vi "Check if File Exists _NOT Folder.vi"(8 "error in (no error)":errorcluster, 11 "path":path) -> (0 "error out":errorcluster, 2 "file exists?":bool, 3 "dup path":path)   [LabVIEW 2021]
doc: "Checks whether a file or folder exists on disk at a specified path. This VI works with standard files and folders as well as files in LLB files."
uses:
  <vilib>/Utility/lvfile.llb/FT_FileTypes.ctl
  <vilib>/Utility/lvfile.llb/NI_FileType.lvlib
  <vilib>/Utility/LVLibp/NI_PackedLibraryUtility.lvlib
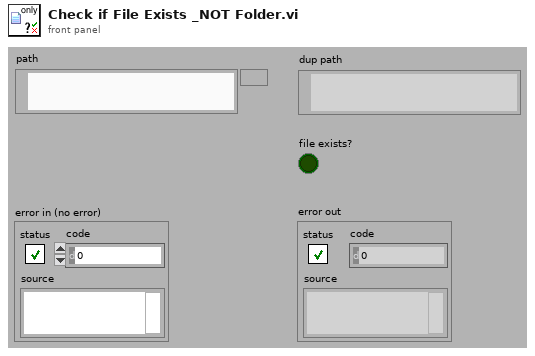
[diagram p1: front panel]
types:
  T1 = typedef "NI_FileType.lvlib/FT_FileTypes.ctl" = enum32{"Invalid file/path", "Unknown type", "Instrument", "Control", "Polymorphic VI", "Project", "Library", "LVClass", "XControl", "XNode", "CIN", "Run-time menu", "Palette menu", "LLB", "Shortcut", "Directory", "Class Private Data Control", "Statechart", "MathScript .m file", "Ladder Diagram", "LVLibp"}
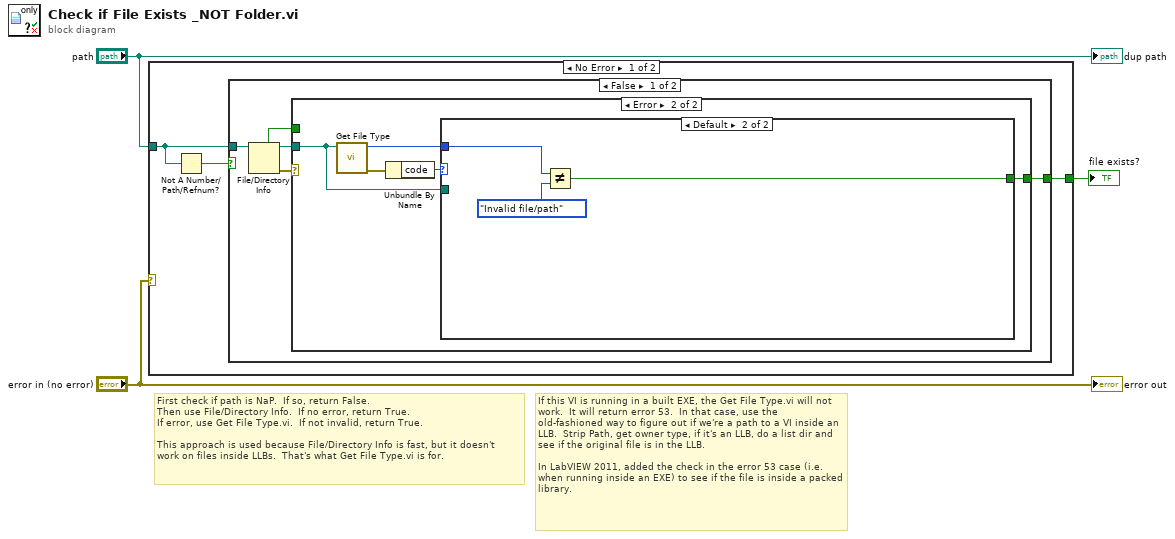
[diagram p0: block diagram]
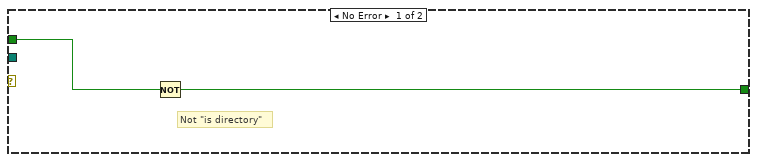
[diagram p2: hidden frame]
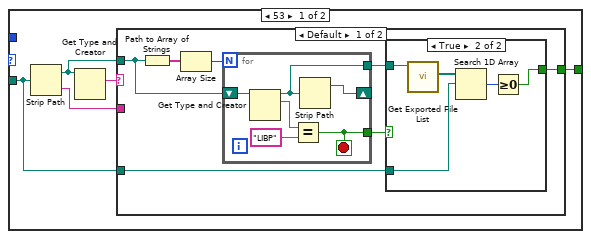
[diagram p3: hidden frame]
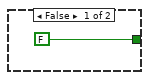
[diagram p4: hidden frame]
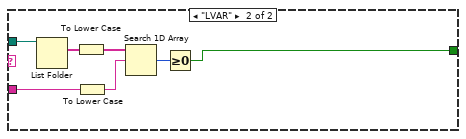
[diagram p5: hidden frame]
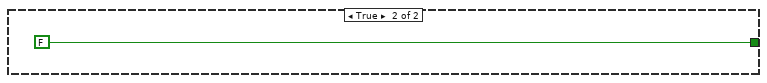
[diagram p6: hidden frame]
diagram:
  # "If this VI is running in a built EXE, the Get File Type.vi will not work.  It will return error 53.  In that case, use the old-fashioned way to figure out if we're a path to a VI inside an LLB.  Strip Path, get owner type, if it's an LLB, do a list dir and see if the original file is in the LLB.\n\nIn LabVIEW 2011, added the check in the error 53 case (i.e. when running inside an EXE) to see if the file is inside a packed library."
  # "First check if path is NaP.  If so, return False.\nThen use File/Directory Info.  If no error, return True.\nIf error, use Get File Type.vi.  If not invalid, return True.\n\nThis approach is used because File/Directory Info is fast, but it doesn't\nwork on files inside LLBs.  That's what Get File Type.vi is for."
  n1 = case shown="No Error" "error in (no error)" {
    tunnel: "path" -> [w5 _]
    tunnel: [w6 _] -> w1
    frame No Error {
      n2 = Not A Number/Path/Refnum?(number/path/refnum=w5) -> (NaN/Path/Refnum?=w4:bool)
      n3 = case shown="False" w4 {
        tunnel: [w9 FALSE] -> w6
        tunnel: w5 -> [w11 _]
        frame False {
          n4 = File/Directory Info(path=w11) -> (path out=w8:path, directory=w7:bool, error out=w10:errorcluster)  [unwired: 1 in, 4 out]
          n5 = case shown="Error" w10 {
            tunnel: [w12 w18] -> w9
            tunnel: w8 -> [_ w14]
            tunnel: w7 -> [w13 _]
            frame No Error {
              # "Not \"is directory\""
              n6 = Not(x=w13) -> (.not. x?=w12:bool)
            }
            frame Error {
              n7 = call <vilib>:"Get File Type.vi"("path"=w14) -> ("error out"=w16:errorcluster, "file type"=w17:T1)  [unwired: 1 in, 8 out]
              n8 = Unbundle By Name(w16) -> ("code"=w15:i32)
              n9 = case shown="Default" w15 {
                tunnel: [w22 w52] -> w18
                tunnel: w17 -> [_ w51]
                tunnel: w14 -> [w19 _]
                frame 53 {
                  n10 = Strip Path(path=w19) -> (stripped path=w20:path, name=w21:string)
                  n11 = Get Type and Creator(7:w20) -> (2:w23:string)  [unwired: 1 in, 3 out]
                  n12 = case shown="Default" w23 {
                    tunnel: [w26 w43] -> w22
                    tunnel: w21 -> [_ w47]
                    tunnel: w20 -> [w28 w49]
                    tunnel: w19 -> [w24 _]
                    frame Default {
                      n13 = Path to Array of Strings(0:w28) -> (2:w30:string[])  [unwired: 1 out]
                      n14 = Array Size(array=w30) -> (size(s)=w29:i32)
                      n15 = for {
                        N: w29 -> [_]
                        shift-right: [w41] -> _
                        shift-left: w28 -> [w42]
                        tunnel: [w38] -> w27
                        tunnel: [w37] -> w25
                        stop <- w38 stop-if-true
                        n16 = Get Type and Creator(7:w42) -> (2:w40:string, 3:w37:path)  [unwired: 1 in, 2 out]
                        n17 = Equal?(x=w40, y="LIBP") -> (x = y?=w38:bool)
                        n18 = Strip Path(path=w37) -> (stripped path=w41:path)  [unwired: 1 out]
                      }
                      n19 = case shown="True" w27 {
                        tunnel: [FALSE w32] -> w26
                        tunnel: w25 -> [_ w36]
                        tunnel: w24 -> [_ w34]
                        frame False {
                        }
                        frame True {
                          n20 = call <vilib>:"Get Exported File List.vi"("packed library path"=w36) -> ("paths"=w35:path[])  [unwired: 8 in, 2 out]
                          n21 = Search 1D Array(1D array=w35, element=w34) -> (index of element=w33:i32)  [unwired: 1 in]
                          n22 = Greater Or Equal To 0?(x=w33) -> (x >= 0?=w32:bool)
                        }
                      }
                    }
                    frame "LVAR" {
                      n23 = List Folder(path=w49) -> (filenames=w48:string[])  [unwired: 1 in, 5 out]
                      n24 = To Lower Case(string=w48) -> (all lower case string=w45:string[])
                      n25 = To Lower Case(string=w47) -> (all lower case string=w46:string)
                      n26 = Search 1D Array(1D array=w45, element=w46) -> (index of element=w44:i32)  [unwired: 1 out]
                      n27 = Greater Or Equal To 0?(x=w44) -> (x >= 0?=w43:bool)
                    }
                  }
                }
                frame Default {
                  n28 = Not Equal?(x=w51, y=FT_FileTypes."Invalid file/path") -> (x != y?=w52:bool)
                }
              }
            }
          }
        }
        frame True {
        }
      }
    }
    frame Error {
    }
  }
  "file exists?" <- w1
  "error out" <- "error in (no error)"
  "dup path" <- "path"
